vi "2023_day08_Task1.vi"() -> ()   [LabVIEW 2021]
panel:
  out "Task 1":i32
  in  "Switch":bool caption="Ex. Data  vs.  User Data"
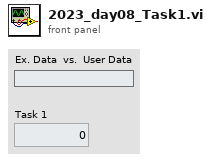
[diagram p1: front panel]
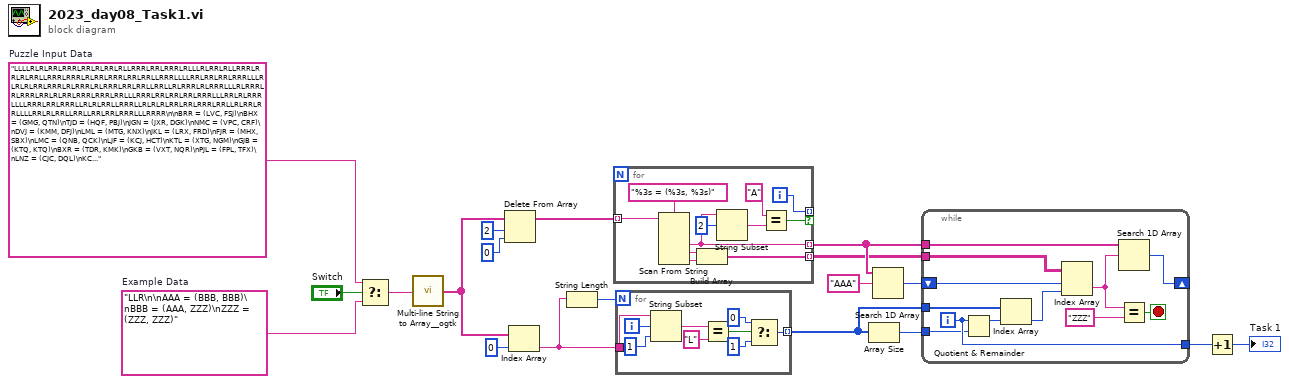
[diagram p0: block diagram]
diagram:
  w1 = "LLR\n\nAAA = (BBB, BBB)\nBBB = (AAA, ZZZ)\nZZZ = (ZZZ, ZZZ)"  # Example Data
  w18 = "LLLLRLRLRRLRRRLRRLRLRRLRLLRRRLRRLRRRLRLLLRLRRLRLLRRRLRRLRLRRLLRRRLRRRLRLRRLRRRLRRLRRLLRRRLLLLRRLRRLRRLRRRLLLRLRLRLRRLRRRLRLRRRLRLRRRLRRLRRLLRRLLRLRRRLRLRRRLLLRLRRRLRLRRRLRRLRLRRLRRRLRRRLRRLLLRRRLRRLRRLRRLRRRLLLRRLRLRRRLLLLRRRLRRLRRRLLRLRLRRLLRRRLLRLRLRLRRLRRLRRRLRRLLRLRRLRRLLLLRRLRLRRLLRRLLRRLRRLRRRLLLRRRR\n\nBRR = (LVC, FSJ)\nBHX = (GMG, QTN)\nTJD = (HQF, PBJ)\nJGN = (JXR, DGK)\nNMC = (VPC, CRF)\nDVJ = (KMM, DFJ)\nLML = (MTG, KNX)\nJKL = (LRX, FRD)\nFJR = (MHX, SBX)\nLMC = (QNB, QCK)\nLJF = (KCJ, HCT)\nKTL = (XTG, NGM)\nGJB = (KTQ, KTQ)\nBXR = (TDR, KMK)\nGKB = (VXT, NQR)\nPJL = (FPL, TFX)\nLNZ = (CJC, DQL)\nKCG = (KDL, LMF)\nPGG = (NDL, XXC)\nPMS = (XQM, DFG)\nCJF = (MCG, RTJ)\nJTH = (PGS, SGZ)\nQBS = (JSC, KMT)\nDQL = (KRR, PBL)\nHSF = (SNP, KJR)\nXVQ = (VQR, HSX)\nQKF = (PBT, XLC)\nDNA = (DQL, CJC)\nLNF = (RVC, TJD)\nMKT = (LDX, CGC)\nBXP = (RGX, TTR)\nSBX = (PGT, JGN)\nJQK = (HDQ, BHQ)\nMHL = (TLX, JDN)\nBBD = (QNJ, BRM)\nMTT = (BVK, DXB)\nFVR = (VLN, PRV)\nRVC = (HQF, PBJ)\nLDX = (LRS, KBV)\nBKF = (PXH, TNB)\nBRM = (XTV, NGH)\nDDL = (JNG, SFF)\nBBT = (BQJ, BCN)\nGPK = (CVK, DDL)\nTLX = (BDN, XNT)\nJHL = (BRX, QBT)\nNTL = (HSR, DJD)\nXBH = (PJX, JQK)\nPPF = (LCT, BJL)\nSFF = (FVR, NFG)\nHNA = (CTC, BSG)\nCNG = (DXM, QFN)\nGML = (NRD, TVN)\nRHH = (NBT, LJH)\nLDM = (DDN, TRN)\nXSK = (PLB, NVJ)\nNCQ = (MDN, XGT)\nFCQ = (HCT, KCJ)\nDRC = (JKL, JNM)\nSHR = (KLX, VLH)\nFTP = (DRN, DKV)\nQBF = (GVS, NXK)\nGXK = (XDK, LVF)\nKMK = (VXV, XCS)\nPKK = (QNJ, BRM)\nNJH = (TKL, PQK)\nBRX = (MNM, HVC)\nVTD = (BJK, LML)\nQVX = (DVJ, DSF)\nGRM = (JCV, SQB)\nRDQ = (HCG, XMB)\nRGX = (FCN, TPD)\nHBH = (FPR, DHX)\nPHM = (JSP, RCR)\nNBT = (FRG, CMJ)\nXRH = (HCB, FBM)\nGMR = (FDJ, NJD)\nMVG = (RDJ, QSD)\nBDL = (JSB, TFN)\nVXT = (MBM, JND)\nTXC = (QDG, LTV)\nSRL = (RRX, NDS)\nSGN = (MPL, CBB)\nHVH = (SLJ, CBC)\nVPC = (CCG, QSJ)\nKCJ = (CKC, TTD)\nRLT = (LLT, VVL)\nRXV = (KXQ, VBR)\nFQS = (STP, BHX)\nSGC = (RLJ, QGB)\nXLX = (HRG, DGV)\nXKV = (QQB, TNQ)\nSLJ = (GTB, MPF)\nPKV = (CQN, THS)\nRPP = (QFT, TNK)\nDKL = (MFC, MFC)\nBCG = (FXM, GPR)\nRFV = (DRC, MPD)\nVVC = (FGN, CVL)\nHQB = (QNT, VVC)\nRRP = (VVC, QNT)\nTRS = (RCM, GHN)\nQBT = (HVC, MNM)\nXKS = (SCC, VXX)\nTPS = (FMH, KFN)\nMTS = (VXT, NQR)\nFXM = (LDM, FQT)\nLNB = (XJV, SJN)\nHVF = (QXC, RBH)\nLSG = (QHM, TSM)\nJMP = (HBH, NQK)\nNGM = (KDP, HHP)\nHCG = (SLR, TSC)\nHGX = (DFG, XQM)\nDLG = (BVN, GMM)\nDJD = (VGP, VML)\nHBT = (XKL, JBQ)\nNVJ = (GKX, PKS)\nCPS = (PKJ, RSV)\nSKN = (NBT, LJH)\nCCK = (TTJ, SLV)\nDXM = (CBN, BXR)\nRJD = (XJH, SKH)\nRDJ = (CNF, TTG)\nPKJ = (BCM, XKC)\nFQL = (SRV, DFC)\nKDS = (MFB, CLQ)\nQKR = (VGD, CXK)\nXXC = (NFD, SPS)\nPSQ = (NJH, BLR)\nBLR = (PQK, TKL)\nLMX = (DGV, HRG)\nGCK = (CSR, CSR)\nGKJ = (JHL, PNN)\nGVS = (TLN, LJX)\nFPR = (JCH, GKD)\nVQV = (DGB, GGN)\nCPF = (VMH, JQQ)\nGKD = (SGF, PHM)\nJNM = (LRX, FRD)\nCXV = (LNF, HGF)\nTNK = (RRD, HKC)\nDXX = (LMC, ZZZ)\nDGG = (PPF, TRR)\nMLH = (TVL, PBR)\nLBC = (LJL, FTR)\nFVQ = (TBC, LKB)\nLTF = (CBC, SLJ)\nTVH = (XMS, GJS)\nSFB = (TTJ, SLV)\nLVF = (MBT, SJB)\nXPP = (QDM, PJL)\nBVK = (RPV, JMP)\nVGD = (MRX, FJR)\nFRD = (XBH, CDN)\nLKM = (CMF, XNS)\nTCJ = (MMS, PGG)\nDHQ = (MTT, BKS)\nHDQ = (GPH, XKH)\nKTJ = (QQT, MKR)\nNMQ = (VFK, VSD)\nRSK = (QDM, PJL)\nXQC = (KFP, HVB)\nLQN = (NGM, XTG)\nTKG = (XDQ, XDQ)\nKBB = (VQR, HSX)\nTQQ = (QDG, LTV)\nSQN = (TDQ, XKV)\nTSM = (TSH, MRP)\nKPH = (THS, CQN)\nHCB = (DVL, RTV)\nMLR = (GHT, NSN)\nBFM = (GCK, SLX)\nGXQ = (QKM, JJL)\nGNF = (HRQ, XTK)\nTRR = (BJL, LCT)\nAAA = (QNB, QCK)\nSDL = (KJX, LSN)\nDKV = (KBB, XVQ)\nRMR = (MQR, CPR)\nMQC = (CBV, SRP)\nPRV = (KDS, FBX)\nGTB = (CCK, SFB)\nSNP = (PXX, SHR)\nNTR = (VHT, KXK)\nMKJ = (DDL, CVK)\nLSQ = (HSF, RMN)\nTTJ = (CBH, QKF)\nDNH = (MVG, JCJ)\nKMM = (KPH, PKV)\nNTT = (RQK, PFK)\nQMF = (BFM, PJB)\nRJB = (RBH, QXC)\nLRS = (MJT, BVM)\nCJG = (RMR, BMN)\nDVQ = (GXM, DDH)\nMFC = (LMC, LMC)\nXTG = (HHP, KDP)\nHKB = (RDQ, TVT)\nPKS = (JQM, DGG)\nBJK = (KNX, MTG)\nTVT = (XMB, HCG)\nJNR = (JHG, JLN)\nVFK = (XKS, QBH)\nNPC = (PKK, BBD)\nPXX = (KLX, VLH)\nXLC = (NST, BXP)\nCBB = (LMX, XLX)\nKLX = (MSH, LCF)\nCLQ = (JNF, JNC)\nTSS = (MKR, QQT)\nSSS = (RMQ, RCS)\nQSD = (TTG, CNF)\nNHG = (DVQ, VNB)\nCTC = (VCN, RJD)\nTHS = (QRH, GPT)\nKDR = (RTK, GKJ)\nNTD = (CGG, SPN)\nGHP = (NCQ, FCD)\nKXQ = (RLS, VRM)\nGNV = (BQJ, BCN)\nDXQ = (QHC, FXN)\nRQB = (FVQ, TNF)\nCNF = (TXC, TQQ)\nBGB = (QQS, LRV)\nZZZ = (QCK, QNB)\nNFM = (MGV, VTD)\nMFD = (DBF, KSN)\nNST = (RGX, TTR)\nXJV = (LGL, LGL)\nTRQ = (TVH, KJL)\nPPV = (CJP, VHH)\nDNV = (DBM, VGJ)\nJBQ = (MHL, RFN)\nHRG = (JFD, VQP)\nRMB = (JKJ, JGJ)\nRGQ = (RSK, XPP)\nKHF = (TJG, KPX)\nHPZ = (BSG, CTC)\nLFJ = (TSN, NMB)\nMBT = (XRC, PJR)\nQFN = (CBN, BXR)\nQSJ = (BRS, BKF)\nXJH = (RSF, VNP)\nGST = (LVF, XDK)\nDDN = (NMS, RLT)\nCXK = (FJR, MRX)\nPHH = (FPB, TCJ)\nXHV = (KTJ, TSS)\nVHT = (NPC, DMG)\nRNL = (NHG, DVN)\nTKL = (KPN, FKX)\nDGB = (GPJ, QMF)\nPNN = (QBT, BRX)\nTBC = (NTR, FKG)\nPGS = (QDT, JQL)\nSLX = (CSR, LNB)\nBVV = (LVC, FSJ)\nJQL = (MLH, GSC)\nPXH = (CJF, CKM)\nLHM = (DSF, DVJ)\nNND = (NTD, DTB)\nMFB = (JNF, JNC)\nTTR = (FCN, TPD)\nHRQ = (JTD, JTD)\nSLR = (TXT, JSN)\nVQP = (XPK, XGB)\nQHM = (MRP, TSH)\nRTJ = (PXB, TLP)\nQQT = (RRL, QHQ)\nCSR = (XJV, XJV)\nCJP = (CJG, HQQ)\nRMC = (MPD, DRC)\nXMS = (LXX, GPN)\nHSR = (VGP, VML)\nMNM = (VSS, QXR)\nSJN = (LGL, LNZ)\nKBV = (MJT, BVM)\nKFN = (NRC, VSG)\nJNC = (RHR, LFJ)\nMPF = (SFB, CCK)\nQVK = (GNK, BCG)\nNJD = (KCG, LDB)\nDBM = (MJG, MFD)\nNKF = (GGN, DGB)\nBCN = (JNR, MHK)\nGNK = (FXM, GPR)\nKMT = (HFC, CPS)\nFDJ = (KCG, LDB)\nLVD = (PHH, QDR)\nFCN = (VDP, MQC)\nQQB = (GJB, GJB)\nPLF = (JNL, HBT)\nQDM = (FPL, TFX)\nGXM = (CLD, NNL)\nMRV = (BCG, GNK)\nLKB = (NTR, FKG)\nTTG = (TQQ, TXC)\nGFD = (VSD, VFK)\nRCS = (KQQ, DNH)\nQXR = (FCQ, LJF)\nHMQ = (RJQ, FQL)\nVCN = (SKH, XJH)\nQQG = (HSR, DJD)\nHGF = (RVC, TJD)\nXMB = (TSC, SLR)\nPJB = (GCK, SLX)\nHFC = (RSV, PKJ)\nJJL = (GXK, GST)\nQTN = (JLV, SGX)\nKDP = (GNV, BBT)\nVRF = (TFN, JSB)\nGPN = (CPF, SRQ)\nTSC = (TXT, JSN)\nCRF = (QSJ, CCG)\nTNF = (TBC, LKB)\nVLH = (LCF, MSH)\nBCV = (JSC, KMT)\nNNL = (KVX, FQS)\nRVT = (HCB, FBM)\nQHC = (QKV, NCJ)\nVDP = (CBV, SRP)\nCBV = (VQV, NKF)\nCMF = (XHV, TPR)\nTRN = (RLT, NMS)\nJSB = (XTH, TRS)\nCFC = (TVT, RDQ)\nKDL = (TKG, TKG)\nTTD = (BBC, GHP)\nKJR = (PXX, SHR)\nMTV = (GVS, NXK)\nBVN = (KDR, PVP)\nDXB = (RPV, JMP)\nFSJ = (QPQ, GML)\nPBJ = (LQN, KTL)\nPXB = (BDL, VRF)\nNDS = (BGB, NGX)\nCBN = (KMK, TDR)\nNFG = (VLN, PRV)\nJTD = (PGS, PGS)\nMKR = (QHQ, RRL)\nJSN = (RFV, RMC)\nCVK = (SFF, JNG)\nFGN = (BVQ, XQC)\nHHF = (RPS, QQF)\nPLB = (PKS, GKX)\nBJB = (QMC, GPG)\nSTP = (QTN, GMG)\nDGK = (RKK, BVT)\nJJM = (VGD, CXK)\nLTS = (QPN, BCL)\nLVC = (QPQ, GML)\nQNB = (GJN, RVB)\nRBH = (HMQ, HPS)\nNQK = (DHX, FPR)\nMRP = (BDT, SGN)\nJQM = (TRR, PPF)\nTSH = (BDT, SGN)\nJLN = (JCC, FCB)\nBRP = (LDX, CGC)\nSJC = (HRQ, HRQ)\nLJL = (BVB, PPV)\nSPN = (SDL, VHM)\nSDM = (DDF, LTS)\nLJH = (FRG, CMJ)\nCMG = (MKD, JGT)\nGPR = (LDM, FQT)\nQPQ = (NRD, TVN)\nJCJ = (RDJ, QSD)\nHSX = (CMG, SHF)\nVML = (RMB, MHC)\nDHX = (JCH, GKD)\nMTG = (FPX, SPD)\nBDT = (MPL, CBB)\nCJC = (PBL, KRR)\nJLS = (LJL, FTR)\nHQF = (LQN, KTL)\nHQQ = (RMR, BMN)\nQMC = (RBP, PXD)\nRPV = (HBH, NQK)\nJHG = (JCC, FCB)\nTPD = (VDP, MQC)\nBHQ = (XKH, GPH)\nXKC = (HDD, GXR)\nRPS = (KJP, KJP)\nQNT = (CVL, FGN)\nJSC = (HFC, CPS)\nKXG = (DTB, NTD)\nCKM = (RTJ, MCG)\nFTD = (KPX, TJG)\nVSD = (XKS, QBH)\nMCG = (TLP, PXB)\nXKH = (HLP, CXV)\nTNB = (CJF, CKM)\nXTH = (RCM, GHN)\nDFN = (GMR, DSS)\nLMF = (TKG, XST)\nFMH = (NRC, VSG)\nXCS = (JTS, GRM)\nGVF = (NDS, RRX)\nCXM = (HGX, PMS)\nVRM = (XJT, DXQ)\nJLV = (QVX, LHM)\nJCH = (PHM, SGF)\nNMS = (VVL, LLT)\nBHS = (XJR, LKM)\nCKC = (BBC, GHP)\nCBH = (XLC, PBT)\nPRL = (QFT, TNK)\nSDF = (VTD, MGV)\nRVB = (MLR, XHT)\nGPT = (PLF, MJX)\nKRR = (RVT, XRH)\nGXR = (BVV, BRR)\nNSN = (RGQ, JMQ)\nKJX = (TCR, MSL)\nPHL = (TSM, QHM)\nMQR = (MTS, GKB)\nXDK = (SJB, MBT)\nNRC = (DGN, BJB)\nJQQ = (LBC, JLS)\nJTS = (JCV, SQB)\nRLJ = (JJM, QKR)\nDTB = (CGG, SPN)\nBRS = (PXH, TNB)\nSRV = (SPC, DNV)\nMNP = (JJL, QKM)\nKTQ = (XSK, XSK)\nFPX = (SJC, GNF)\nVBR = (VRM, RLS)\nKSN = (HQB, RRP)\nRJQ = (SRV, DFC)\nBKS = (BVK, DXB)\nBVB = (VHH, CJP)\nXTK = (JTD, JTH)\nPBT = (BXP, NST)\nPVP = (RTK, GKJ)\nQPN = (BCV, QBS)\nQQF = (KJP, HPZ)\nQRH = (PLF, MJX)\nGHS = (BKN, TPS)\nRCM = (MNP, GXQ)\nDCT = (DDF, LTS)\nJLC = (HGX, PMS)\nVNC = (XSK, CXZ)\nBQJ = (MHK, JNR)\nSHF = (JGT, MKD)\nFXN = (QKV, NCJ)\nFPB = (PGG, MMS)\nJGJ = (KXG, NND)\nVBM = (PSQ, QKN)\nGKX = (DGG, JQM)\nDSF = (KMM, DFJ)\nCMJ = (GPK, MKJ)\nNCJ = (SDM, DCT)\nMKD = (GQG, DHQ)\nCFZ = (RQB, SHH)\nRQK = (DKL, DKL)\nXGT = (HPQ, VRQ)\nSRP = (NKF, VQV)\nBSG = (VCN, RJD)\nXRC = (NFM, SDF)\nDVL = (SRL, GVF)\nHVB = (HXS, MLD)\nMPD = (JNM, JKL)\nJSP = (PHL, LSG)\nBCR = (XJR, LKM)\nPQK = (KPN, FKX)\nFCD = (XGT, MDN)\nMDL = (JLC, CXM)\nFBX = (CLQ, MFB)\nVNP = (RGM, GHS)\nHMK = (RMN, HSF)\nSJB = (PJR, XRC)\nJFD = (XPK, XGB)\nHHP = (GNV, BBT)\nTVN = (VBM, KJN)\nDMG = (PKK, BBD)\nRGM = (BKN, TPS)\nTRF = (KXQ, VBR)\nXHT = (NSN, GHT)\nDFJ = (KPH, PKV)\nKJP = (CTC, BSG)\nLLT = (NTS, LVD)\nRMN = (SNP, KJR)\nGSC = (TVL, PBR)\nRSV = (XKC, BCM)\nTLP = (VRF, BDL)\nGGN = (GPJ, QMF)\nXJR = (CMF, XNS)\nGQG = (BKS, MTT)\nJPN = (MRV, QVK)\nRSF = (RGM, GHS)\nQQS = (DLG, JPV)\nDGV = (VQP, JFD)\nJDN = (XNT, BDN)\nLMA = (QDT, JQL)\nQDG = (QGC, DTX)\nHDD = (BVV, BRR)\nRRD = (CNG, XLJ)\nQBH = (VXX, SCC)\nGPH = (HLP, CXV)\nCVN = (MRV, QVK)\nRLS = (XJT, DXQ)\nQKN = (NJH, BLR)\nNRD = (VBM, KJN)\nNMB = (HVF, RJB)\nXNT = (RXV, TRF)\nXNS = (XHV, TPR)\nSGX = (LHM, QVX)\nNTS = (PHH, QDR)\nSPS = (LTF, HVH)\nKPX = (BCR, BHS)\nGNM = (RPS, RPS)\nCXZ = (NVJ, PLB)\nVVL = (LVD, NTS)\nVTC = (NHG, DVN)\nPXD = (BHH, SSS)\nTVL = (MKT, BRP)\nTPR = (KTJ, TSS)\nMJX = (JNL, HBT)\nBKN = (FMH, KFN)\nMBM = (BVC, FTP)\nRTV = (GVF, SRL)\nGPG = (PXD, RBP)\nKXK = (DMG, NPC)\nJPV = (GMM, BVN)\nLXP = (VPC, CRF)\nRMQ = (DNH, KQQ)\nDRN = (KBB, XVQ)\nMMS = (XXC, NDL)\nGMG = (SGX, JLV)\nMJT = (KHF, FTD)\nXJT = (QHC, FXN)\nJMQ = (XPP, RSK)\nQCS = (TVH, KJL)\nBVC = (DRN, DKV)\nSPC = (DBM, VGJ)\nSHH = (TNF, FVQ)\nVGA = (PLB, NVJ)\nRKK = (JPN, CVN)\nSCC = (TRQ, QCS)\nCDN = (JQK, PJX)\nVSS = (LJF, FCQ)\nJNF = (LFJ, RHR)\nVGP = (MHC, RMB)\nVGJ = (MJG, MFD)\nQGC = (RHH, SKN)\nRKJ = (KTQ, VNC)\nDTX = (SKN, RHH)\nHPQ = (VDR, SGC)\nCCG = (BRS, BKF)\nVLN = (FBX, KDS)\nBHH = (RMQ, RCS)\nBBC = (FCD, NCQ)\nJCV = (GNM, GNM)\nTNQ = (GJB, RKJ)\nQNJ = (NGH, XTV)\nGHT = (RGQ, JMQ)\nLJX = (CFC, HKB)\nTLN = (HKB, CFC)\nPFK = (DKL, LFL)\nPJR = (SDF, NFM)\nJNG = (NFG, FVR)\nPJX = (BHQ, HDQ)\nVHH = (CJG, HQQ)\nRTK = (PNN, JHL)\nXGB = (MLN, SQN)\nJCC = (NQX, NTT)\nBVT = (CVN, JPN)\nHPS = (RJQ, FQL)\nTCR = (DFN, RHS)\nLLA = (SHH, RQB)\nNGX = (QQS, LRV)\nSLV = (CBH, QKF)\nBMN = (CPR, MQR)\nXKL = (RFN, MHL)\nCGG = (VHM, SDL)\nKJN = (PSQ, QKN)\nLDB = (KDL, LMF)\nSPD = (SJC, GNF)\nVDR = (RLJ, QGB)\nDDF = (QPN, BCL)\nKQQ = (MVG, JCJ)\nDSS = (FDJ, NJD)\nNFD = (HVH, LTF)\nGPJ = (BFM, PJB)\nLGL = (DQL, CJC)\nTDQ = (QQB, TNQ)\nRCR = (PHL, LSG)\nSKH = (VNP, RSF)\nDGN = (QMC, GPG)\nNGH = (RNL, VTC)\nTSN = (HVF, RJB)\nMGV = (LML, BJK)\nQHQ = (LXP, NMC)\nKJL = (GJS, XMS)\nRBP = (BHH, SSS)\nQDR = (FPB, TCJ)\nRHR = (NMB, TSN)\nNXK = (LJX, TLN)\nFCB = (NQX, NTT)\nTFN = (TRS, XTH)\nMJG = (KSN, DBF)\nBVQ = (KFP, HVB)\nGMM = (PVP, KDR)\nMDN = (VRQ, HPQ)\nLTV = (DTX, QGC)\nLRV = (DLG, JPV)\nMHC = (JKJ, JGJ)\nDFC = (DNV, SPC)\nLXV = (SHH, RQB)\nPBL = (RVT, XRH)\nBDN = (RXV, TRF)\nJKJ = (KXG, NND)\nMSH = (MTV, QBF)\nNDL = (SPS, NFD)\nFKG = (VHT, KXK)\nPBR = (MKT, BRP)\nVSG = (BJB, DGN)\nRRX = (BGB, NGX)\nNQR = (JND, MBM)\nMRX = (MHX, SBX)\nDVN = (DVQ, VNB)\nHKC = (CNG, XLJ)\nPGT = (JXR, DGK)\nDBF = (HQB, RRP)\nFRG = (GPK, MKJ)\nDFG = (NMQ, GFD)\nQDT = (MLH, GSC)\nKVX = (STP, BHX)\nLCT = (MDL, KCL)\nLSN = (TCR, MSL)\nTXT = (RMC, RFV)\nMXM = (LXV, CFZ)\nTJG = (BHS, BCR)\nBCM = (GXR, HDD)\nFKX = (NTL, QQG)\nSRQ = (JQQ, VMH)\nBCL = (BCV, QBS)\nLRX = (CDN, XBH)\nRHS = (DSS, GMR)\nCLD = (FQS, KVX)\nXLJ = (DXM, QFN)\nKCL = (CXM, JLC)\nHXS = (PRL, RPP)\nJND = (BVC, FTP)\nVQR = (SHF, CMG)\nVNB = (DDH, GXM)\nQGB = (JJM, QKR)\nCVL = (BVQ, XQC)\nRFN = (JDN, TLX)\nFBM = (DVL, RTV)\nTFX = (LSQ, HMK)\nXQM = (NMQ, GFD)\nBJL = (KCL, MDL)\nFTR = (PPV, BVB)\nKNX = (FPX, SPD)\nMHK = (JHG, JLN)\nTDR = (XCS, VXV)\nHVC = (VSS, QXR)\nQXC = (HPS, HMQ)\nRRL = (NMC, LXP)\nMLD = (PRL, RPP)\nLCF = (MTV, QBF)\nVXV = (JTS, GRM)\nXTV = (RNL, VTC)\nLFL = (MFC, DXX)\nCBC = (GTB, MPF)\nCQN = (GPT, QRH)\nDDH = (NNL, CLD)\nGHN = (GXQ, MNP)\nJGT = (DHQ, GQG)\nHCT = (CKC, TTD)\nQCK = (GJN, RVB)\nSGF = (JSP, RCR)\nMPL = (XLX, LMX)\nXDQ = (LXV, LXV)\nMLN = (TDQ, XKV)\nSGZ = (JQL, QDT)\nVRQ = (SGC, VDR)\nFPL = (LSQ, HMK)\nSQB = (GNM, HHF)\nMHX = (PGT, JGN)\nQFT = (HKC, RRD)\nLXX = (CPF, SRQ)\nCPR = (GKB, MTS)\nHLP = (LNF, HGF)\nGJS = (GPN, LXX)\nQKV = (DCT, SDM)\nXST = (XDQ, MXM)\nVXX = (QCS, TRQ)\nKFP = (HXS, MLD)\nMSL = (RHS, DFN)\nNQX = (RQK, PFK)\nCGC = (LRS, KBV)\nFQT = (TRN, DDN)\nVMH = (LBC, JLS)\nVHM = (LSN, KJX)\nJXR = (BVT, RKK)\nKPN = (QQG, NTL)\nQKM = (GST, GXK)\nJNL = (XKL, JBQ)\nBVM = (KHF, FTD)\nXPK = (SQN, MLN)\nGJN = (MLR, XHT)"  # Puzzle Input Data
  n1 = Select(t=w18, s="Switch", f=w1) -> (s? t:f=w17:string)
  n2 = call <userlib>:"Multi-line String to Array__ogtk.vi"("string"=w17) -> ("lines"=w14:string[])
  n3 = Delete From Array(array=w14, length=2, index=0) -> (array with subset deleted=w5:string[])  [unwired: 1 out]
  n4 = Index Array(array=w14, index=0) -> (element=w12:string)
  n5 = String Length(string=w12) -> (length=w11:i32)
  n6 = for {
    tunnel: w5 -> [w30] mode=indexing
    tunnel: [w29] -> w3 mode=indexing
    tunnel: [w22] -> w4 mode=indexing
    tunnel: [w21] -> _ mode=indexing if=w20
    i -> [w21]
    n7 = Scan From String(format string="%3s = (%3s, %3s)", input string=w30) -> (output 1=w22:string, output 2=w26:string, output 3=w27:string)  [unwired: 5 in, 3 out]
    n8 = Build Array(w26, w27) -> (w29:string[])
    n9 = String Subset(string=w22, offset (0)=2) -> (substring=w24:string)  [unwired: 1 in]
    n10 = Equal?(x="A", y=w24) -> (x = y?=w20:bool)
  }
  n11 = for {
    N: w11 -> [_]
    tunnel: w12 -> [w39]
    tunnel: [w31] -> w2 mode=indexing
    i -> [w38]
    n12 = String Subset(string=w39, offset (0)=w38, length (rest)=1 ("length (rest)")) -> (substring=w32:string)
    n13 = Equal?(x=w32, y="L") -> (x = y?=w34:bool)
    n14 = Select(t=0, s=w34, f=1) -> (s? t:f=w31:i32)
  }
  n15 = Array Size(array=w2) -> (size(s)=w6:i32)
  n16 = Search 1D Array(1D array=w4, element="AAA") -> (index of element=w8:i32)  [unwired: 1 in]
  n17 = while {
    tunnel: w2 -> [w51]
    tunnel: w4 -> [w49]
    tunnel: w3 -> [w47]
    shift-right: [w45] -> _
    shift-left: w8 -> [w46]
    tunnel: [w42] -> w10
    tunnel: w6 -> [w41]
    i -> [w42]
    stop <- w43 stop-if-true
    n18 = Quotient & Remainder(x=w42, y=w41) -> (x-y*floor(x/y)=w50:i32)  [unwired: 1 out]
    n19 = Index Array(array=w51, index=w50) -> (element=w48:i32)
    n20 = Index Array(array=w47, index (row)=w46, index (col)=w48) -> (element=w44:string)
    n21 = Search 1D Array(1D array=w49, element=w44) -> (index of element=w45:i32)  [unwired: 1 in]
    n22 = Equal?(x=w44, y="ZZZ") -> (x = y?=w43:bool)
  }
  n23 = Increment(x=w10) -> (x+1=→"Task 1":i32)
